vi "F Dwf Analog In Status Data16.vi"(6 "cdData":i32, 7 "idxData":i32, 8 "error in (no error)":errorcluster, 9 "rgu16Data":i16, 10 "idxChannel":i32, 11 "hdwf":i32) -> (0 "error out":errorcluster, 1 "rgu16Data out":i16, 3 "function return":i32)   [LabVIEW 2021, in "Olasdwf.lvlib"]
doc: "DWFAPI int FDwfAnalogInStatusData16(HDWF hdwf, int idxChannel, short *rgu16Data, int idxData, int cdData);"
uses:
  Olasdwf.lvlib
  Windows/System32/dwf.dll
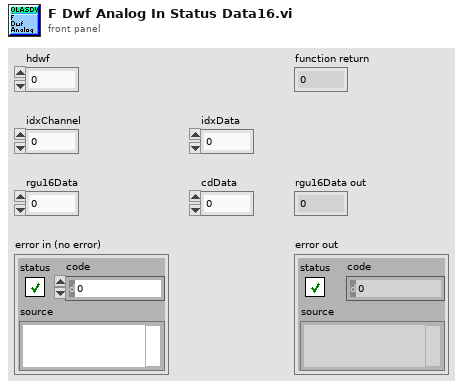
[diagram p1: front panel]
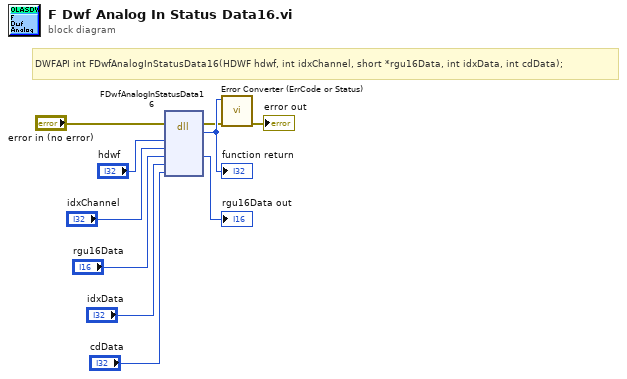
[diagram p0: block diagram]
diagram:
  # "DWFAPI int FDwfAnalogInStatusData16(HDWF hdwf, int idxChannel, short *rgu16Data, int idxData, int cdData);"
  n1 = dll-call lib="/Windows/System32/dwf.*" fn="FDwfAnalogInStatusData16"(error in="error in (no error)", "hdwf"="hdwf", "idxChannel"="idxChannel", "rgu16Data"="rgu16Data", "idxData"="idxData", "cdData"="cdData") -> (error out=w2:errorcluster, w10:i32, "rgu16Data"=→"rgu16Data out":i16)  [unwired: 6 in, 1 out]
  "function return" <- w10
  n2 = call "Error Converter (ErrCode or Status).vi"("error in (no error)"=w2, "error code"=w10) -> ("error out"=→"error out":errorcluster)  [unwired: 9 in]
